vi "Match-Value Image (ARGB).vi"(8 "error in (no error)":errorcluster, 9 "Value":T1={"Alpha"=255, "RGB"=0}, 10 "Match Destination":T2, 11 "ARGB Image Source":T3) -> (0 "error out":errorcluster, 3 "Match Destination (duplicate)":T2)   [LabVIEW 2020, in "image.lvlib"]
uses:
  image.lvlib
  ARGB Image.ctl
  Greyscale Image.ctl
  ARGB Colour.ctl
  5701baee-35e2-4306-9a77-a9fdbb5b3a7f.vi
  common/Module Path.vi
  <vilib>/Utility/error.llb/Error Cluster From Error Code.vi
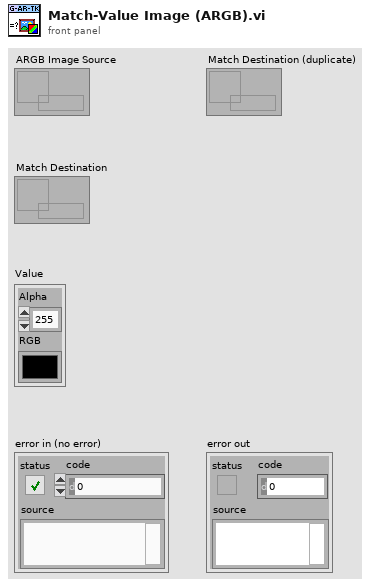
[diagram p1: front panel]
types:
  T1 = typedef "image.lvlib/ARGB Colour.ctl" = cluster{"Alpha":u8, "RGB":u32}
  T2 = typedef "image.lvlib/Greyscale Image.ctl" = refnum<data-value>
  T3 = typedef "image.lvlib/ARGB Image.ctl" = refnum<data-value>
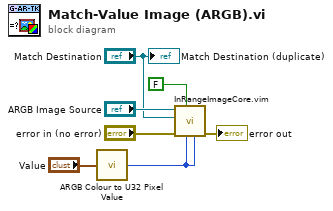
[diagram p0: block diagram]
diagram:
  n1 = call "ARGB Colour to U32 Pixel Value.vi"("ARGB Colour"="Value") -> ("U32 Colour"=w1:u32)
  n2 = call "InRangeImageCore.vim"("Upper"=w1, "Lower"=w1, "IgnoreAlpha"=FALSE, "error in (no error)"="error in (no error)", "In-Range-Result"="Match Destination", "Src"="ARGB Image Source") -> ("error out"=→"error out":errorcluster)  [unwired: 5 in]
  "Match Destination (duplicate)" <- "Match Destination"
